vi "Write Data.vi"(8 "error in (no error)":errorcluster, 10 "Data":dbl[](array[numeric]), 11 "Dbl Array in":refnum<class "Dbl Array.lvclass">) -> (0 "error out":errorcluster, 3 "Dbl Array out":refnum<class "Dbl Array.lvclass">)   [LabVIEW 2012, in "Base Data Class.lvlib" / "Dbl Array.lvclass"]
uses:
  Dbl Array.lvclass
  Dbl Array.lvclass/Dbl Array.ctl
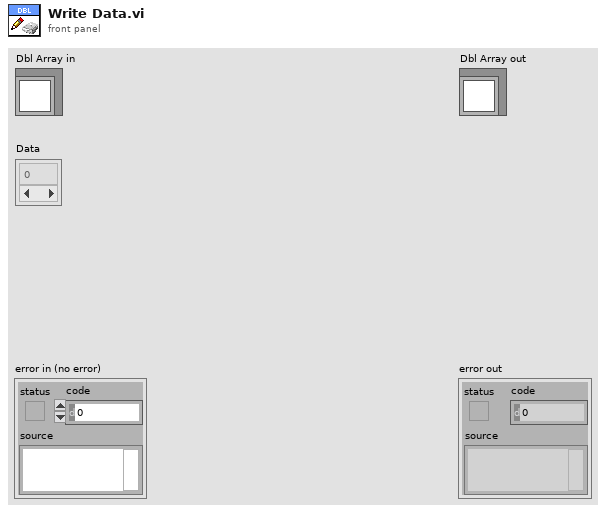
[diagram p1: front panel]
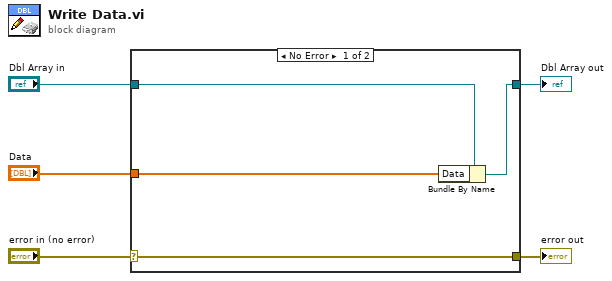
[diagram p0: block diagram]
diagram:
  n1 = case shown="No Error" "error in (no error)" {
    selector: "error in (no error)" -> [w9 w10]
    tunnel: [w9 w10] -> w4
    tunnel: [w7 w11] -> w2
    tunnel: "Dbl Array in" -> [w8 w11]
    tunnel: "Data" -> [w6 _]
    frame No Error {
      n2 = Bundle By Name(cluster=w8, "Data"=w6) -> (w7:refnum<class "Dbl Array.lvclass">)
    }
    frame Error {
    }
  }
  "error out" <- w4
  "Dbl Array out" <- w2
